vi "Write File Path.vi"(8 "error in (no error)":errorcluster, 10 "File Path":path, 11 "Tree Data File in":refnum<class "Tree Data File.lvclass">) -> (0 "error out":errorcluster, 3 "Tree Data File out":refnum<class "Tree Data File.lvclass">)   [LabVIEW 2019, in "Tree Data File.lvclass"]
uses:
  Tree Data File.lvclass
  Tree Data File.lvclass/Tree Data File.ctl
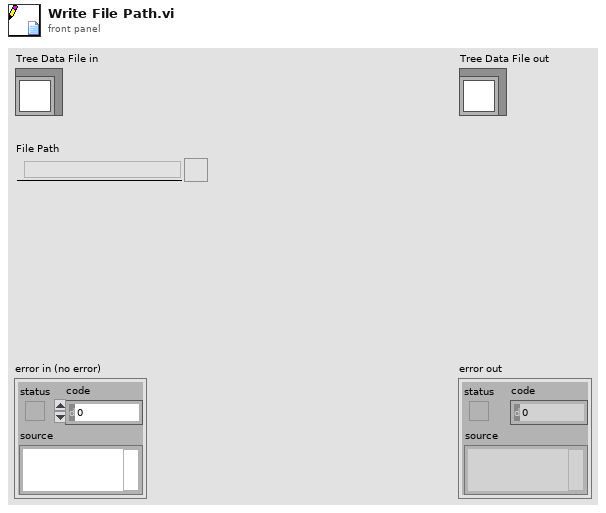
[diagram p1: front panel]
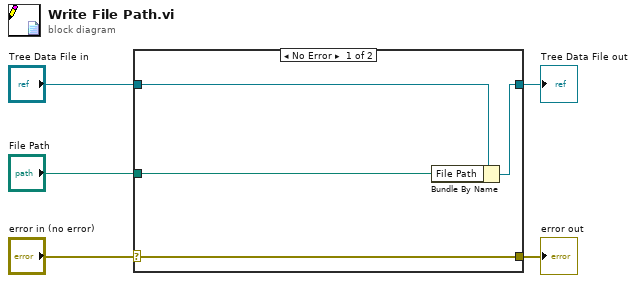
[diagram p0: block diagram]
diagram:
  n1 = case shown="No Error" "error in (no error)" {
    selector: "error in (no error)" -> [w9 w10]
    tunnel: [w9 w10] -> w4
    tunnel: [w7 w11] -> w2
    tunnel: "Tree Data File in" -> [w8 w11]
    tunnel: "File Path" -> [w6 _]
    frame No Error {
      n2 = Bundle By Name(cluster=w8, "File Path"=w6) -> (w7:refnum<class "Tree Data File.lvclass">)
    }
    frame Error {
    }
  }
  "error out" <- w4
  "Tree Data File out" <- w2
